vi "Main.vi"() -> ()   [LabVIEW 2020, in "1039_mod.lvlib"]
doc: "This template is based off of the Queued Message Handler design pattern and the Queued Message Handler project template that ships with LabVIEW.\n\nThe main difference is that the queue is private to this module and communication between modules is performed via Broadcast and Request events.\n\nRequest events are wrapped in public API methods and are handled in the Event Handling Loop (EHL) of this VI. Any module can register for Broadcast events sent by this module. The EHL generates messages based on user interface actions.\n\nThe Message Handling Loop (MHL) processes messages generated by the EHL, or by other messages. The messages are string values, so new messages can be added easily to the Message Cases case structure in the MHL. Each message cluster can also provide an optional value for Message Data, which is a variant that can be converted to whatever message-specific data is required.\n_____\nBased on Delacor QMH Project Template 4.2.1.64."
uses:
  1039_mod.lvlib
  <vilib>/Delacor/Delacor QMH/Libraries/Module Admin_class/Delacor_lib_QMH_Module Admin.lvclass
  thcd_controls/ctrl_chn_thcd.ctl
  thcd_controls/ctrl_uom_thcd.ctl
  thcd_controls/ctrl_gid_thcd.ctl
  Module Data--cluster.ctl
  <vilib>/Delacor/Delacor QMH/Libraries/Message Queue_class/Delacor_lib_QMH_Message Queue.lvclass/Delacor_lib_QMH_Message Queue.ctl
  Stop Argument--cluster.ctl
  <vilib>/Delacor/Delacor QMH/Libraries/Module Admin_class/Delacor_lib_QMH_Module Admin.lvclass/Delacor_lib_QMH_Module Admin.ctl
  Initialize Communication Argument--cluster.ctl
  Initialize Instrument Argument--cluster.ctl
  Configure Instrument Argument--cluster.ctl
  Perform Measurement Argument--cluster.ctl
  Perform Measurement (Reply Payload)--cluster.ctl
  <vilib>/Utility/miscctls.llb/LVPointTypeDef.ctl
  <vilib>/Delacor/Delacor QMH/Libraries/Message Queue_class/Delacor_lib_QMH_Enqueue Message (Single).vi
  <vilib>/Delacor/Delacor QMH/Libraries/Module Admin_class/Delacor_lib_QMH_Get External Launch.vi
  <vilib>/Utility/error.llb/Error Cluster From Error Code.vi
  thcd_commands/thcd_set_uom.vi
  thcd_commands/thcd_set_gid.vi
  <vilib>/ErrorRing/Error Ring.xnode
  <vilib>/Delacor/Delacor QMH/Libraries/Message Queue_class/Delacor_lib_QMH_Message Queue.lvclass
panel:
  in  "module_id":u16
  in  "thcd_gid":T1
  in  "thcd_ch":T2
  in  "thcd_uom":T3
  out "thcd_res_1":T4
  in  "dev_baud_rate":u32(ring)=19200 items=["9.6KHz"=9600, "19.2KHz"=19200]
  in  "module_port":refnum<visa-resource-name>
  in  "Simulate MHL Error":bool
  in  "Simulate EHL Error":bool
  out "error out":errorcluster
  in  "Module Admin":refnum<class "Delacor_lib_QMH_Module Admin.lvclass">
  out "Status":string
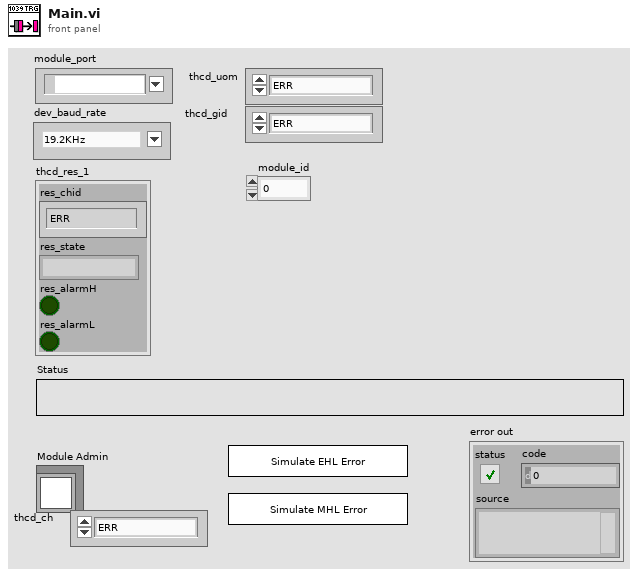
[diagram p1: front panel]
types:
  T1 = typedef "ctrl_gid_thcd.ctl" = enum16{"ERR", "1", "2", "C3H6O_1", "C2H3N", "C2H2", "Air", "C3H4_1", "NH3", "Ar", "AsH3", "C6H6", "BCl3", "BF3", "Br2", "15", "16", "CBrF3", "C4H10_1", "19", "C4H8_1", "CO2", "CS2", "CO", "CCl4", "COS", "Cl2", "ClF3", "28", "29", "CHCl3", "31", "32", "C4H8_2", "C2N2", "ClCN", "C4H8_3", "C3H6", "H22", "B2H6", "40", "R21", "42", "43", "44", "45", "46", "47", "48", "C2H7N_1", "C2H6O_1", "C2H6S_1", "C4H6_1", "C2H6", "54", "55", "C2H6O_2", "C4H6_2", "C2H7N_2", "C8H10", "60", "61", "C2H5F", "C2H4", "64", "65", "C2H4O", "C2H4N", "68", "C2H6S_2", "F2", "CH2O", "CCl3F", "73", "CClF3", "CF4", "76", "CHF3", "78", "C4H4O", "He", "C3HF7", "HMDS", "83", "C6H14", "C6F6", "C6H12_1", "N2H4", "H2", "HBr", "HCl", "CHN", "HF", "HI", "H2Se", "H2S", "C4H10_2", "97", "C4H8_4", "C5H12_1", "C3H8O_1", "101", "C2H2O", "Kr", "CH4", "CH4O", "106", "C3H4_2", "CH5N", "CH3Br", "CH3Cl", "C7H14", "C3H9N", "C3H8O_2", "C3H8S", "CH3F", "116", "CH3I", "CH4S", "C6H12_2", "C3H6O_2", "Ne", "NO", "N2", "NO2", "N2O4", "NF3", "127", "NOCl", "N2O", "C5H12_2", "C8H18", "O2", "F2O", "O3", "B5H9", ""}
  T2 = typedef "ctrl_chn_thcd.ctl" = enum8{"ERR", "1", "2", "3", "4"}
  T3 = typedef "ctrl_uom_thcd.ctl" = enum16{"ERR", "SCCM", "SLM", "%", "V", "MV", "CNT", "NLM", "SLS", "NLS", "SLH", "NLH", "SMLM", "NMLM", "SMLS", "NMLS", "SMLH", "NMLH", "NCCM", "SCCS", "NCCS", "SCCH", "NCCH", "SCFM", "NCFM", "SCFS", "NCFS", "SCFH", "NCFH", "SCMM", "NCMM", "SCMS", "NCMS", "SCMH", "NCMH", "SCIM", "NCIM", "SCIS", "NCIS", "SCIH", "NCIH", "LBM", "LBS", "LBH", "KgM", "KgS", "KgH", "GRM", "GMS", "GRH", "MolM", "MolS", "MolH", "KMolM", "KMolS", "KMolH", "W", "BPS", "Sec", "Min", "Hrs", "WH", "Torr", "Bar", "Pa", "inH2O", "PSIA", "PSIG"}
  T4 = cluster{"res_chid":T2, "res_state":string, "res_alarmH":bool, "res_alarmL":bool}
  T5 = typedef "1039_mod.lvlib/Request Events--cluster.ctl" = cluster{"Stop Module":refnum<user-event>, "Show Panel":refnum<user-event>, "Hide Panel":refnum<user-event>, "Get Module Execution Status":refnum<user-event>, "Show Diagram":refnum<user-event>, "Initialize Communication":refnum<user-event>, "Initialize Instrument":refnum<user-event>, "Configure Instrument":refnum<user-event>, "Perform Measurement":refnum<user-event>}
  T6 = typedef "1039_mod.lvlib/Module Data--cluster.ctl" = cluster{"Status":string}
  T7 = enum32{"invalid lock state", "Not Locked", "Locked (No Password)", "Password-protected"}
  T8 = typedef "1039_mod.lvlib/Stop Argument--cluster.ctl" = cluster{"Origin":string, "Exit via Stop Module Req?":bool, "Wait for Module to stop?":bool}
  T9 = typedef "1039_mod.lvlib/Initialize Communication Argument--cluster.ctl" = cluster{"com_source":enum16{"request argument", "configuration file", "module setting"}, "com_port":refnum<visa-resource-name>}
  T10 = typedef "1039_mod.lvlib/Initialize Instrument Argument--cluster.ctl" = cluster{"status_type":enum16{"status", "value"}}
  T11 = typedef "1039_mod.lvlib/Configure Instrument Argument--cluster.ctl" = cluster{"config_type":enum16{"module setting", "configuration file"}}
  T12 = typedef "1039_mod.lvlib/Perform Measurement Argument--cluster.ctl" = cluster{"read_source":enum16{"request argument", "configuration file", "module setting"}, "Wait Notifier":refnum<notifier>, "wait for reply":bool}
  T13 = typedef "LVPointTypeDef.ctl" = cluster{"Horizontal":i16, "Vertical":i16}
  T14 = enum32{"Invalid", "Standard", "Closed", "Hidden", "Minimized", "Maximized"}
  T15 = typedef "1039_mod.lvlib/Perform Measurement (Reply Payload)--cluster.ctl" = cluster{"module_id":u16, "timestamp":dbl, "value":dbl[], "Perform Measurement_error":errorcluster}
  T16 = enum16{"request argument", "configuration file", "module setting"}
  T17 = cluster{"res_chid":T2, "res_val":dbl, "res_uom":string, "res_gid":string}
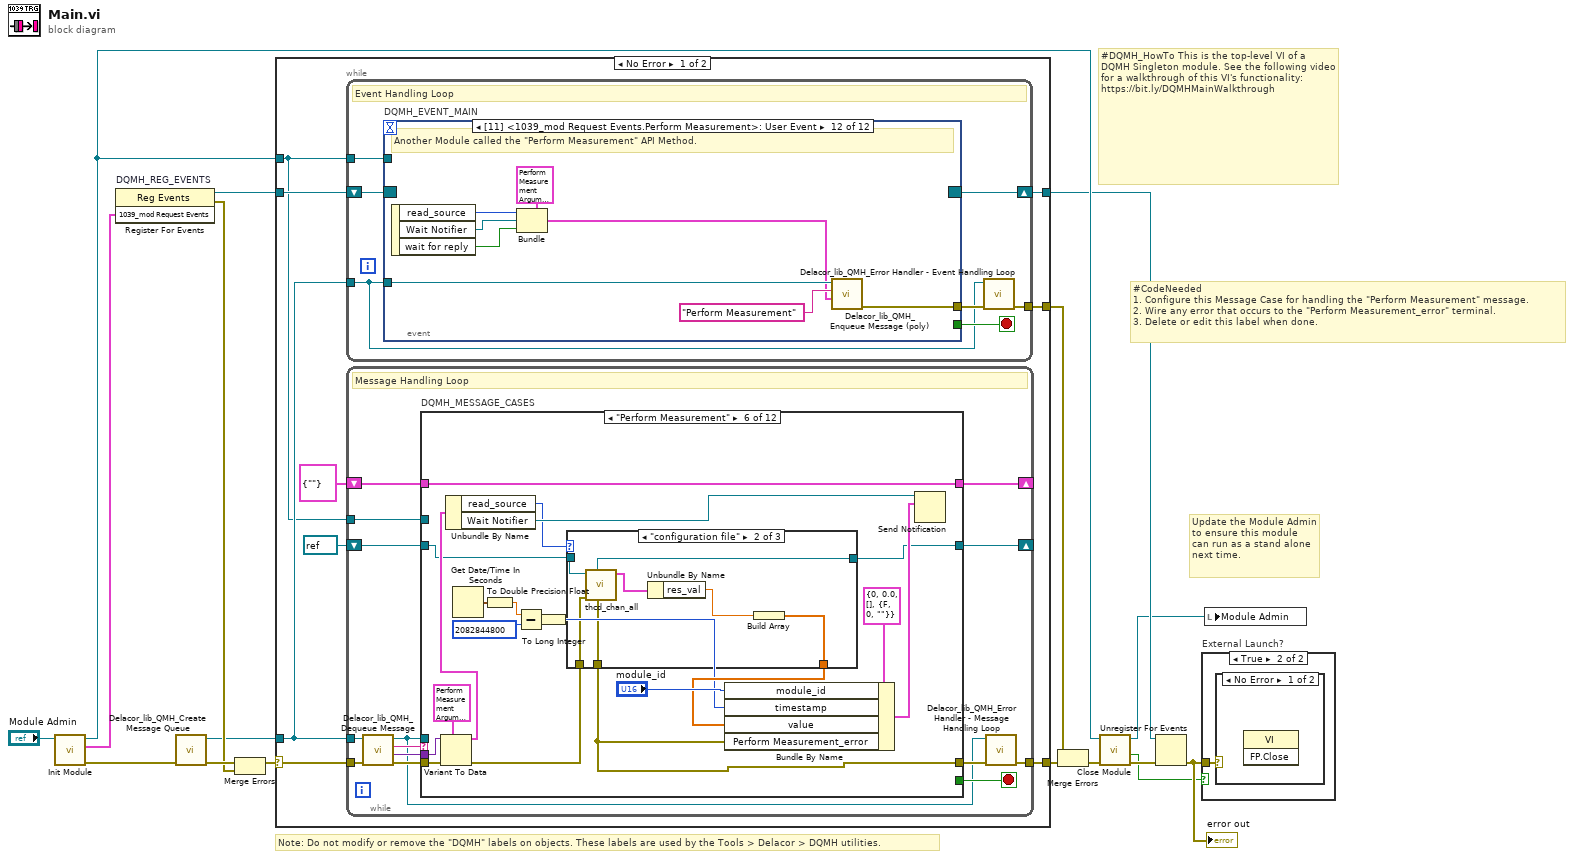
[diagram p0: block diagram]
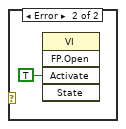
[diagram p3: hidden frame]
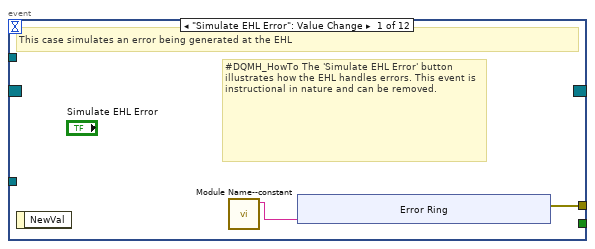
[diagram p4: hidden frame]
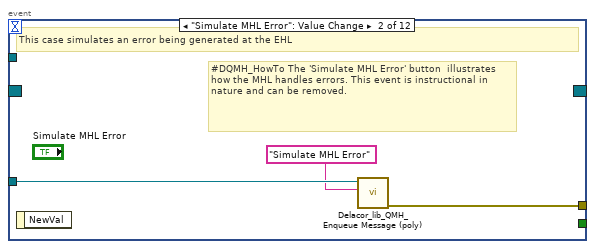
[diagram p5: hidden frame]
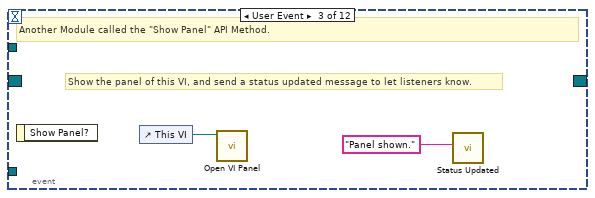
[diagram p6: hidden frame]
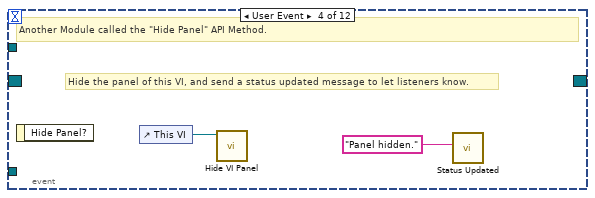
[diagram p7: hidden frame]
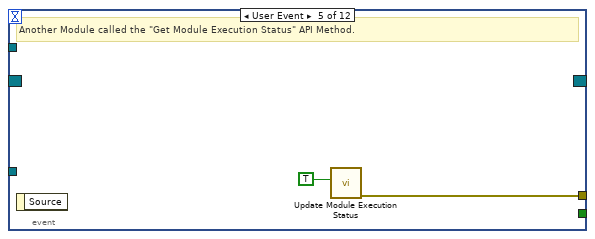
[diagram p8: hidden frame]
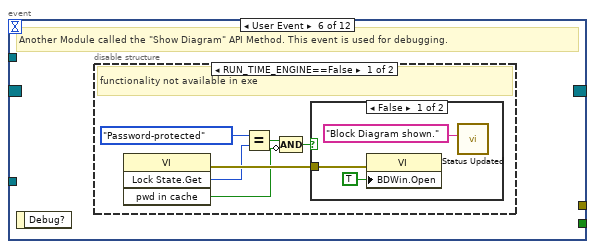
[diagram p9: hidden frame]
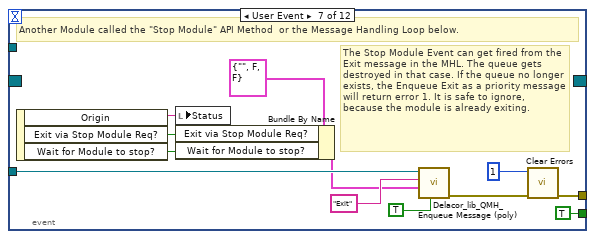
[diagram p12: hidden frame]
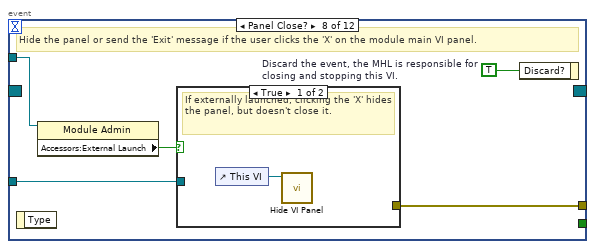
[diagram p13: hidden frame]
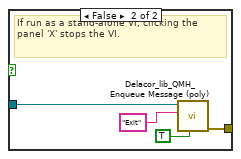
[diagram p14: hidden frame]
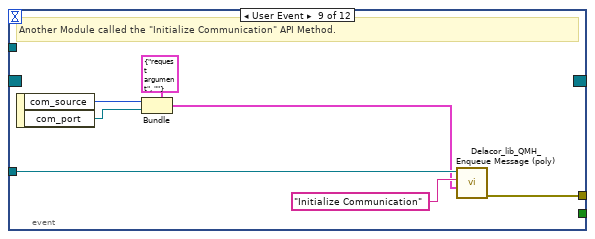
[diagram p15: hidden frame]
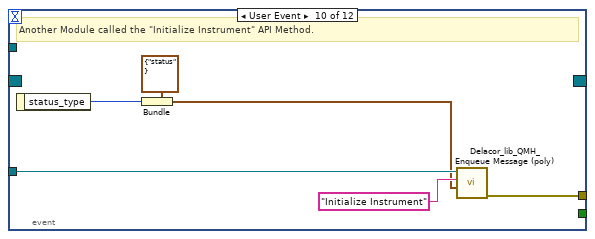
[diagram p16: hidden frame]
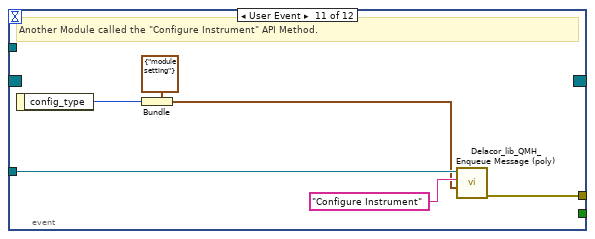
[diagram p17: hidden frame]
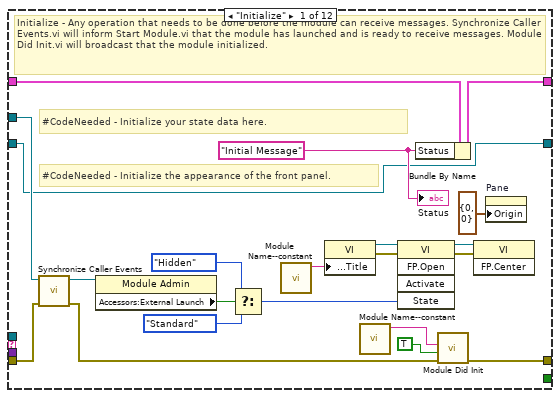
[diagram p18: hidden frame]
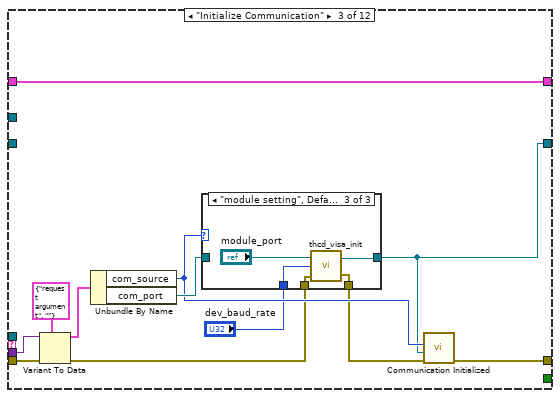
[diagram p20: hidden frame]
diagram:
  # "#CodeNeeded\n1. Configure this Message Case for handling the \"Perform Measurement\" message.\n2. Wire any error that occurs to the \"Perform Measurement_error\" terminal.\n3. Delete or edit this label when done."
  # "#DQMH_HowTo This is the top-level VI of a DQMH Singleton module. See the following video for a walkthrough of this VI's functionality: https://bit.ly/DQMHMainWalkthrough"
  # "Note: Do not modify or remove the \"DQMH\" labels on objects. These labels are used by the Tools > Delacor > DQMH utilities."
  # "Update the Module Admin to ensure this module can run as a stand alone next time."
  n1 = call "Init Module.vi"("Singleton Module Admin in"="Module Admin") -> ("error out"=w16:errorcluster, "1039_mod Request Events"=w5:T5, "Singleton Module Admin out"=w8:refnum<class "Delacor_lib_QMH_Module Admin.lvclass">)  [unwired: 8 in]
  n2 = register-events "DQMH_REG_EVENTS"(w5) -> (reference out=w6:refnum<event-registration>, error out=w9:errorcluster)  [unwired: 2 in]
  n3 = call <vilib>:"Delacor_lib_QMH_Create Message Queue.vi"("error in"=w16) -> ("error out"=w11:errorcluster, "Message Queue"=w4:refnum<class "Delacor_lib_QMH_Message Queue.lvclass">)  [unwired: 9 in]
  n4 = Merge Errors(w11, w9) -> (w10:errorcluster)
  n5 = case shown="No Error" w10 {
    selector: w10 -> [w24 w342]
    tunnel: [w26 w342] -> w17
    tunnel: [w23 w339] -> w7
    tunnel: w6 -> [w21 w339]
    tunnel: w4 -> [w20 _]
    tunnel: [w25 _] -> w14
    tunnel: w8 -> [w19 w335]
    frame No Error {
      n6 = while {
        tunnel: w20 -> [w27]
        shift-right: [w30] -> w23
        shift-left: w21 -> [w31]
        tunnel: [w32] -> w25
        tunnel: w19 -> [w28]
        stop <- w29 stop-if-true
        # "Event Handling Loop"
        n7 = event "DQMH_EVENT_MAIN" shown="[11] <1039_mod Request Events.Perform Measurement>: User Event" {
          selector: w31 -> [_ _ _ _ _ _ _ _ _ _ _ _]
          dyn-events: [_ _ _ _ _ _ _ _ _ _ _ _] -> w30
          timeout: _ -> [_ _ _ _ _ _ _ _ _ _ _ _]
          tunnel: [_ _ _ _ _ _ TRUE ("Discard?") _ _ _ _ _] -> w29
          tunnel: w27 -> [_ w44 _ _ _ _ w68 w75 w89 w95 w101 w109]
          tunnel: [w35 w45 _ _ w51 _ w71 w77 w83 w90 w96 w102] -> w33
          tunnel: w28 -> [_ _ _ _ _ _ _ w74 _ _ _ _]
          event "Simulate EHL Error": Value Change {
            # "#DQMH_HowTo The 'Simulate EHL Error' button  illustrates how the EHL handles errors. This event is instructional in nature and can be removed."
            # "This case simulates an error being generated at the EHL"
            n8 = event-data() -> ()  [unwired: 1 in, 1 out]
            n9 = call "Module Name--constant.vi"() -> ("Module Name"=w34:string)  [unwired: 11 in]
            n10 = xnode "Error Ring"("parameter 0"=w34) -> ("error out"=w35:errorcluster)
          }
          event "Simulate MHL Error": Value Change {
            # "#DQMH_HowTo The 'Simulate MHL Error' button  illustrates how the MHL handles errors. This event is instructional in nature and can be removed."
            # "This case simulates an error being generated at the EHL"
            n11 = event-data() -> ()  [unwired: 1 in, 1 out]
            n12 = call-poly <vilib>:"Delacor_lib_QMH_Enqueue Message (poly).vi"("Message"="Simulate MHL Error", "Message Queue in"=w44) -> ("error out"=w45:errorcluster)  [unwired: 8 in, 1 out]
          }
          event User Event {
            # "Show the panel of this VI, and send a status updated message to let listeners know."
            # "Another Module called the \"Show Panel\" API Method."
            n13 = event-data() -> ()  [unwired: 1 in, 1 out]
            n14 = control-ref of="This VI"() -> (w47:refnum<vi>)
            n15 = call "Open VI Panel.vi"("VI"=w47) -> ()  [unwired: 10 in, 1 out]
            n16 = call "Status Updated.vi"("Status"="Panel shown." ("format string")) -> ()  [unwired: 10 in, 1 out]
          }
          event User Event {
            # "Hide the panel of this VI, and send a status updated message to let listeners know."
            # "Another Module called the \"Hide Panel\" API Method."
            n17 = event-data() -> ()  [unwired: 1 in, 1 out]
            n18 = control-ref of="This VI"() -> (w49:refnum<vi>)
            n19 = call "Hide VI Panel.vi"("VI"=w49) -> ()  [unwired: 10 in, 1 out]
            n20 = call "Status Updated.vi"("Status"="Panel hidden." ("format string")) -> ()  [unwired: 10 in, 1 out]
          }
          event User Event {
            # "Another Module called the \"Get Module Execution Status\" API Method."
            n21 = event-data() -> ()  [unwired: 1 in, 1 out]
            n22 = call "Update Module Execution Status.vi"("Running?"=TRUE) -> ("error out"=w51:errorcluster)  [unwired: 10 in]
          }
          event User Event {
            # "Another Module called the \"Show Diagram\" API Method. This event is used for debugging."
            n23 = event-data() -> ()  [unwired: 1 in, 1 out]
            n24 = disable-structure shown="RUN_TIME_ENGINE==False" {
              frame condition #0 (active) {
                # "functionality not available in exe"
                n25 = invoke class="VI" method="Lock State.Get"() -> (error out=w57:errorcluster, "Get Lock State"=w56:T7, "pwd in cache"=w53:bool)  [unwired: 4 in, 1 out]
                n26 = Equal?(x=T7."Password-protected", y=w56) -> (x = y?=w54:bool)
                n27 = Compound Arithmetic op=AND(w54, invert w53) -> (w52:bool)
                n28 = case shown="False" w52 {
                  tunnel: w57 -> [w60 _]
                  frame False {
                    n29 = property class="VI"(error in=w60, "BDWin.Open"=TRUE ("Block Diagram Window:Open")) -> ()  [unwired: 1 in, 2 out]
                    n30 = call "Status Updated.vi"("Status"="Block Diagram shown." ("format string")) -> ()  [unwired: 10 in, 1 out]
                  }
                  frame True {
                    # "Password-protected VI, and the password is not in the cache. Do not show the diagram."
                  }
                }
              }
              frame condition #1 {
              }
            }
          }
          event User Event {
            # "The Stop Module Event can get fired from the Exit message in the MHL. The queue gets destroyed in that case. If the queue no longer exists, the Enqueue Exit as a priority message will return error 1. It is safe to ignore, because the module is already exiting."
            # "Another Module called the \"Stop Module\" API Method  or the Message Handling Loop below."
            n31 = event-data() -> ("Origin"=w67:string, "Exit via Stop Module Req?"=w63:bool, "Wait for Module to stop?"=w62:bool)  [unwired: 1 in]
            n32 = local write "Status"(w67) -> ()
            n33 = Bundle By Name(cluster=T8 {"Origin"="", "Exit via Stop Module Req?"=FALSE, "Wait for Module to stop?"=FALSE} ("Stop Argument"), "Exit via Stop Module Req?"=w63, "Wait for Module to stop?"=w62) -> (w61:T8)
            n34 = call-poly <vilib>:"Delacor_lib_QMH_Enqueue Message (poly).vi"("Priority Message? (F)"=TRUE, "Message Data"=w61, "Message"="Exit", "Message Queue in"=w68) -> ("error out"=w72:errorcluster)  [unwired: 6 in, 1 out]
            n35 = call <vilib>:"Clear Errors.vi"("error in (no error)"=w72, "specific error code to clear (0: all)"=1) -> ("error out"=w71:errorcluster)  [unwired: 4 in, 1 out]
          }
          event Panel Close? {
            w76 = TRUE  # Discard the event, the MHL is responsible for closing and stopping this VI.
            # "Hide the panel or send the 'Exit' message if the user clicks the 'X' on the module main VI panel."
            n36 = event-data() -> ()  [unwired: 1 in, 1 out]
            n37 = property class="Module Admin"(reference=w74) -> ("Accessors:External Launch"=w73:bool)  [unwired: 1 in, 2 out]
            n38 = case shown="True" w73 {
              tunnel: w75 -> [_ w81]
              tunnel: [_ w82] -> w77
              frame True {
                # "If externally launched, clicking the 'X' hides the panel, but doesn't close it."
                n39 = control-ref of="This VI"() -> (w78:refnum<vi>)
                n40 = call "Hide VI Panel.vi"("VI"=w78) -> ()  [unwired: 10 in, 1 out]
              }
              frame False {
                # "If run as a stand-alone VI, clicking the panel 'X' stops the VI."
                n41 = call-poly <vilib>:"Delacor_lib_QMH_Enqueue Message (poly).vi"("Priority Message? (F)"=TRUE, "Message"="Exit", "Message Queue in"=w81) -> ("error out"=w82:errorcluster)  [unwired: 7 in, 1 out]
              }
            }
            n42 = event-data("Discard?"=w76) -> ()  [unwired: 1 in, 1 out]
          }
          event User Event {
            # "Another Module called the \"Initialize Communication\" API Method."
            n43 = event-data() -> ("com_source"=w85:T16, "com_port"=w84:refnum<visa-resource-name>)  [unwired: 1 in]
            n44 = Bundle(cluster=T9 {"com_source"=enum."request argument", "com_port"=""} ("Initialize Communication Argument"), "com_source"=w85, "com_port"=w84) -> (w86:T9)
            n45 = call-poly <vilib>:"Delacor_lib_QMH_Enqueue Message (poly).vi"("Message Data"=w86, "Message"="Initialize Communication", "Message Queue in"=w89) -> ("error out"=w83:errorcluster)  [unwired: 7 in, 1 out]
          }
          event User Event {
            # "Another Module called the \"Initialize Instrument\" API Method."
            n46 = event-data() -> ("status_type"=w91:enum16{"status", "value"})  [unwired: 1 in]
            n47 = Bundle(cluster=T10 {"status_type"=enum."status"} ("Initialize Instrument Argument"), "status_type"=w91) -> (w92:T10)
            n48 = call-poly <vilib>:"Delacor_lib_QMH_Enqueue Message (poly).vi"("Message Data"=w92, "Message"="Initialize Instrument", "Message Queue in"=w95) -> ("error out"=w90:errorcluster)  [unwired: 7 in, 1 out]
          }
          event User Event {
            # "Another Module called the \"Configure Instrument\" API Method."
            n49 = event-data() -> ("config_type"=w97:enum16{"module setting", "configuration file"})  [unwired: 1 in]
            n50 = Bundle(cluster=T11 {"config_type"=enum."module setting"} ("Configure Instrument Argument"), "config_type"=w97) -> (w98:T11)
            n51 = call-poly <vilib>:"Delacor_lib_QMH_Enqueue Message (poly).vi"("Message Data"=w98, "Message"="Configure Instrument", "Message Queue in"=w101) -> ("error out"=w96:errorcluster)  [unwired: 7 in, 1 out]
          }
          event User Event {
            # "Another Module called the \"Perform Measurement\" API Method."
            n52 = event-data() -> ("read_source"=w105:T16, "Wait Notifier"=w104:refnum<notifier>, "wait for reply"=w103:bool)  [unwired: 1 in]
            n53 = Bundle(cluster=T12 {"read_source"=enum."request argument", "Wait Notifier"=refnum, "wait for reply"=FALSE} ("Perform Measurement Argument"), "read_source"=w105, "Wait Notifier"=w104, "wait for reply"=w103) -> (w106:T12)
            n54 = call-poly <vilib>:"Delacor_lib_QMH_Enqueue Message (poly).vi"("Message Data"=w106, "Message"="Perform Measurement", "Message Queue in"=w109) -> ("error out"=w102:errorcluster)  [unwired: 7 in, 1 out]
          }
        }
        n55 = call-dynamic "Delacor_lib_QMH_Error Handler - Event Handling Loop.vi"("error in"=w33, "Message Queue in"=w27) -> ("dup error in"=w32:errorcluster)  [unwired: 8 in, 1 out]
      }
      n56 = while {
        tunnel: w20 -> [w114]
        shift-right: [w118] -> _
        shift-left: T6 {"Status"=""} ("Data Cluster") -> [w119]
        tunnel: w24 -> [w122]
        tunnel: [w120] -> w26
        tunnel: w19 -> [w112]
        shift-right: [w111] -> _
        shift-left: refnum<visa-resource-name> refnum ("module_port") -> [w110]
        stop <- w117 stop-if-true
        # "Message Handling Loop"
        n57 = call-dynamic "Delacor_lib_QMH_Dequeue Message.vi"("error in"=w122, "Message Queue in"=w114) -> ("error out"=w121:errorcluster, "Message Data"=w115:variant, "Message"=w116:string, "Message Queue out"=w113:refnum<class "Delacor_lib_QMH_Message Queue.lvclass">)  [unwired: 6 in]
        n58 = case "DQMH_MESSAGE_CASES" shown="\"Perform Measurement\"" w116 {
          selector: w116 -> [_ _ _ _ _ _ _ _ _ _ _ w322]
          tunnel: w113 -> [_ _ _ _ _ _ _ _ _ w290 w313 _]
          tunnel: w121 -> [w142 w147 w159 w181 w210 w246 w270 w273 w279 w297 w319 w324]
          tunnel: [w140 w147 w153 w170 w194 w232 w269 w273 w278 w293 w316 w325] -> w123
          tunnel: w119 -> [w131 w146 w158 w180 w209 w245 w268 w272 w276 w292 w312 w323]
          tunnel: [w130 w146 w158 w180 w209 w245 w268 w272 w276 w292 w312 w323] -> w118
          tunnel: [_ _ _ _ _ _ _ _ _ _ w311 _] -> w117
          tunnel: w115 -> [_ _ w157 w179 w208 w244 _ _ _ w291 w310 _]
          tunnel: w112 -> [w132 _ _ _ _ _ _ _ _ w289 w305 _]
          tunnel: [w124 w145 w148 w174 w200 w236 w267 w271 w274 w287 w304 w320] -> w111
          tunnel: w110 -> [w124 w145 _ w175 w204 w237 w267 w271 w274 w287 w304 w320]
          frame "Initialize" {
            w125 = "Initial Message" ("Initial Message")
            # "#CodeNeeded - Initialize the appearance of the front panel."
            # "#CodeNeeded - Initialize your state data here."
            # "Initialize - Any operation that needs to be done before the module can receive messages. Synchronize Caller Events.vi will inform Start Module.vi that the module has launched and is ready to receive messages. Module Did Init.vi will broadcast that the module initialized."
            n59 = call "Synchronize Caller Events.vi"("error in (no error)"=w142, "Singleton Module Admin in"=w132) -> ("error out"=w141:errorcluster, "Singleton Module Admin out"=w127:refnum<class "Delacor_lib_QMH_Module Admin.lvclass">)  [unwired: 8 in]
            n60 = property class="Module Admin"(reference=w127) -> ("Accessors:External Launch"=w136:bool)  [unwired: 1 in, 2 out]
            n61 = Select(t=T14."Hidden" ("State"), s=w136, f=T14."Standard" ("State")) -> (s? t:f=w133:T14)
            n62 = call "Module Name--constant.vi"() -> ("Module Name"=w139:string)  [unwired: 11 in]
            n63 = property class="VI"("Front Panel.Title"=w139) -> (reference out=w138:refnum<vi>, error out=w144:errorcluster)  [unwired: 2 in]
            n64 = call "Module Name--constant.vi"() -> ("Module Name"=w128:string)  [unwired: 11 in]
            n65 = invoke class="VI" method="FP.Open"(reference=w138, error in=w144, "State"=w133) -> (reference out=w137:refnum<vi>, error out=w143:errorcluster)  [unwired: 2 in, 3 out]
            n66 = Bundle By Name(cluster=w131, "Status"=w125) -> (w130:T6)
            n67 = call "Module Did Init.vi"("error in (no error)"=w141, "Initialized?"=TRUE, "Origin"=w128) -> ("error out"=w140:errorcluster)  [unwired: 8 in]
            n68 = invoke class="VI" method="FP.Center"(reference=w137, error in=w143) -> ()  [unwired: 1 in, 3 out]
            n69 = property on="Pane" class="Pane"("Origin"=T13 {"Horizontal"=0, "Vertical"=0}) -> ()  [unwired: 2 in, 2 out]
            "Status" <- w125
          }
          frame "--- Module Specific ---" {
            # "Separator -- The following cases handle messages specific to this Module."
          }
          frame "Initialize Communication" {
            n70 = Variant To Data(error in=w159, type=T9 {"com_source"=enum."request argument", "com_port"=""} ("Initialize Communication Argument"), Variant=w157) -> (data=w155:T9, error out=w150:errorcluster)
            n71 = Unbundle By Name(w155) -> ("com_source"=w152:T16, "com_port"=w154:refnum<visa-resource-name>)
            n72 = case shown="\"module setting\", Default" w152 {
              tunnel: [w161 refnum<visa-resource-name> refnum ("module_port") w167] -> w148
              tunnel: w154 -> [w161 _ _]
              tunnel: "dev_baud_rate" -> [_ _ w166]
              tunnel: w150 -> [w160 w162 w165]
              tunnel: [w160 w162 w164] -> w149
              frame "request argument" {
              }
              frame "configuration file" {
              }
              frame "module setting", Default {
                n73 = call "thcd_visa_init.vi"("err_in"=w165, "Serial Settings:Baud Rate"=w166, "thcd_visa"="module_port") -> ("err_out"=w164:errorcluster, "thcd_visa"=w167:refnum<visa-resource-name>)
              }
            }
            n74 = call "Communication Initialized.vi"("error in (no error)"=w149, "com_port"=w148, "com_source"=w152) -> ("error out"=w153:errorcluster)  [unwired: 8 in]
          }
          frame "Initialize Instrument" {
            n75 = Variant To Data(error in=w181, type=T10 {"status_type"=enum."status"} ("Initialize Instrument Argument"), Variant=w179) -> (data=w177:T10, error out=w173:errorcluster)
            n76 = Unbundle By Name(w177) -> ("status_type"=w176:enum16{"status", "value"})
            n77 = case shown="\"status\", Default" w176 {
              tunnel: w175 -> [w189 w192]
              tunnel: [w188 w192] -> w174
              tunnel: w173 -> [w187 w191]
              tunnel: [w184 w191] -> w171
              tunnel: [w183 T4 {"res_chid"=enum."1", "res_state"="ok", "res_alarmH"=TRUE, "res_alarmL"=TRUE} ("thcd_res_1")] -> w172
              tunnel: [w182 TRUE ("thcd_st")] -> w169
              frame "status", Default {
                n78 = call "thcd_chan_stat.vi"("err_in"=w187, "thcd_b2r"=u32 300, "thcd_delay"=u32 300, "thcd_visa"=w189) -> ("thcd_res_1"=w183:T4, "thcd_st"=w182:bool, "err_out"=w184:errorcluster, "thcd_visa"=w188:refnum<visa-resource-name>)  [unwired: 4 out]
              }
              frame "value" {
              }
            }
            "thcd_res_1" <- w172
            n79 = call "Instrument Initialized.vi"("error in (no error)"=w171, "instr_status"=w169) -> ("error out"=w170:errorcluster)  [unwired: 9 in]
          }
          frame "Configure Instrument" {
            n80 = Variant To Data(error in=w210, type=T11 {"config_type"=enum."module setting"} ("Configure Instrument Argument"), Variant=w208) -> (data=w206:T11, error out=w201:errorcluster)
            n81 = Unbundle By Name(w206) -> ("config_type"=w205:enum16{"module setting", "configuration file"})
            n82 = case shown="\"configuration file\"" w205 {
              tunnel: w204 -> [w221 w226]
              tunnel: "thcd_uom" -> [w212 w224]
              tunnel: "thcd_ch" -> [w218 _]
              tunnel: w201 -> [w217 w225]
              tunnel: [w216 w226] -> w200
              tunnel: "thcd_gid" -> [w213 w223]
              tunnel: [w214 w225] -> w196
              tunnel: [w212 w224] -> w198
              tunnel: [w213 w223] -> w197
              tunnel: [w211 TRUE ("thcd_st")] -> w195
              frame "module setting", Default {
                n83 = call-poly "thcd_setters.vi"("thcd_delay"=u32 500, "err_in"=w217, "thcd_val"=w212, "thcd_ch"=w218, "thcd_visa"=w221) -> ("err_out"=w215:errorcluster, "thcd_visa"=w219:refnum<visa-resource-name>)  [unwired: 1 in, 2 out]
                n84 = call-poly "thcd_setters.vi"("err_in"=w215, "thcd_val"=w213, "thcd_ch"=w218, "thcd_visa"=w219) -> ("err_out"=w214:errorcluster, "thcd_st"=w211:bool, "thcd_visa"=w216:refnum<visa-resource-name>)  [unwired: 2 in, 1 out]
              }
              frame "configuration file" {
              }
            }
            n85 = call "Instrument Configured.vi"("config_stat"=w195, "error in (no error)"=w196, "config_set2"=w197, "config_set1"=w198) -> ("error out"=w194:errorcluster)  [unwired: 7 in]
          }
          frame "Perform Measurement" {
            n86 = Variant To Data(error in=w246, type=T12 {"read_source"=enum."request argument", "Wait Notifier"=refnum, "wait for reply"=FALSE} ("Perform Measurement Argument"), Variant=w244) -> (data=w242:T12, error out=w233:errorcluster)
            n87 = Unbundle By Name(w242) -> ("read_source"=w238:T16, "Wait Notifier"=w241:refnum<notifier>)
            n88 = Get Date/Time In Seconds() -> (seconds since 1Jan1904=w229:timestamp)
            n89 = To Double Precision Float(number=w229) -> (double precision float=w231:dbl)
            n90 = Subtract(x=w231, y=2082844800 ("01Jan1970, UTC")) -> (x-y=w230:dbl)
            n91 = To Long Integer(number=w230) -> (32bit integer=w227:i32)
            n92 = case shown="\"configuration file\"" w238 {
              tunnel: w237 -> [w248 w256 w258]
              tunnel: [w248 w255 w258] -> w236
              tunnel: [dbl[] [] w250 w259] -> w234
              tunnel: [w247 w254 w257] -> w232
              tunnel: w233 -> [w247 w253 w257]
              frame "request argument", Default {
              }
              frame "configuration file" {
                n93 = call "thcd_chan_all.vi"("err_in"=w253, "thcd_visa"=w256) -> ("thcd_res_1"=w252:T17, "err_out"=w254:errorcluster, "thcd_visa"=w255:refnum<visa-resource-name>)  [unwired: 5 in, 2 out]
                n94 = Unbundle By Name(w252) -> ("res_val"=w251:dbl)
                n95 = Build Array(w251) -> (w250:dbl[])
              }
              frame "module setting" {
                n96 = for {
                  N: 3 -> [_]
                  tunnel: [w261] -> w259 mode=indexing
                  i -> [w264]
                  n97 = Random Number (0-1)() -> (number: 0 to 1=w266:dbl)
                  n98 = Increment(x=w264) -> (x+1=w263:i32)
                  n99 = Multiply(x=10.0, y=w263) -> (x*y=w262:dbl)
                  n100 = Add(x=w266, y=w262) -> (x+y=w261:dbl)
                }
              }
            }
            n101 = Bundle By Name(cluster=T15 {"module_id"=0, "timestamp"=0.0, "value"=[], "Perform Measurement_error"={"status"=FALSE, "code"=0, "source"=""}} ("Perform Measurement (Reply Payload)"), "module_id"="module_id", "timestamp"=w227, "value"=w234, "Perform Measurement_error"=w232) -> (w240:T15)
            n102 = Send Notification(notification=w240, notifier=w241) -> ()  [unwired: 1 in, 2 out]
          }
          frame "---Copy This Frame---" {
            # "Duplicate this frame when creating new messages.  Change this comment in the duplicated frame to describe this message."
            n103 = Merge Errors(w270) -> (w269:errorcluster)
          }
          frame "--- Exit and Error Handling---" {
            # "Separator - The following cases handle errors and exit messages."
          }
          frame "Simulate MHL Error" {
            # "#DQMH_HowTo The 'Simulate MHL Error' button  illustrates how the MHL handles errors. This event is instructional in nature and can be removed."
            # "Simulate an error occurring at the MHL"
            n104 = call "Module Name--constant.vi"() -> ("Module Name"=w275:string)  [unwired: 11 in]
            n105 = xnode "Error Ring"("parameter 0"=w275) -> ("error out"=w277:errorcluster)
            n106 = Merge Errors(w279, w277) -> (w278:errorcluster)
          }
          frame "Error" {
            # "#CodeRecommended - If you ever change the name of this \"Error\" message, you'll need to update the name in the Check Loop Error.vi as well."
            # "#CodeRecommended - If the module is running in standalone mode (External Launch = FALSE), this code will pop up an error dialog and call the 'Exit' message if an error occurs. Add more fine-grained error handling here."
            # "Error - Check the error message data and respond accordingly. This message is sent by the \"Error Handler\" VIs at the end of each loop in this application."
            n107 = property class="Module Admin"(reference=w289) -> ("Accessors:External Launch"=w288:bool)  [unwired: 1 in, 2 out]
            n108 = Variant To Data(error in=w297, type=errorcluster {"status"=FALSE, "code"=0, "source"=""} ("error constant"), Variant=w291) -> (data=w298:errorcluster, error out=w295:errorcluster)
            n109 = call "Error Reported.vi"("Error"=w298) -> ()  [unwired: 10 in, 1 out]
            n110 = case shown="False" w288 {
              tunnel: [w303 _] -> w294
              tunnel: w290 -> [w301 _]
              tunnel: w298 -> [w302 _]
              frame False {
                # "If the module is running standalone, then pop up an error dialog and call the \"Exit\" message."
                n111 = call <vilib>:"Simple Error Handler.vi"("error in (no error)"=w302) -> ()  [unwired: 4 in, 5 out]
                n112 = call-poly <vilib>:"Delacor_lib_QMH_Enqueue Message (poly).vi"("Priority Message? (F)"=TRUE, "Message"="Exit", "Message Queue in"=w301) -> ("error out"=w303:errorcluster)  [unwired: 7 in, 1 out]
              }
              frame True {
                # "If the module was launched externally, calling the Error Reported broadcast VI is the only action performed by the \"Error\" message. The module's caller can then process the error appropriately."
              }
            }
            n113 = Merge Errors(w295, w294) -> (w293:errorcluster)
            n114 = local write "error out"(w293) -> ()
          }
          frame "Exit" {
            w309 = 91  # 91: not all Exit messages will have an argument
            w311 = TRUE  # Stop the VI
            # "Release the message queue reference"
            # "#CodeNeeded - Add any required cleanup code here"
            # "Exit - Exit the application."
            n115 = Variant To Data(error in=w319, type=T8 {"Origin"="", "Exit via Stop Module Req?"=FALSE, "Wait for Module to stop?"=FALSE} ("Stop Argument"), Variant=w310) -> (data=w307:T8, error out=w315:errorcluster)
            n116 = call <vilib>:"Clear Errors.vi"("error in (no error)"=w315, "specific error code to clear (0: all)"=w309) -> ("error out"=w318:errorcluster)  [unwired: 4 in, 1 out]
            n117 = control-ref of="This VI"() -> (w306:refnum<vi>)
            n118 = call-dynamic "Delacor_lib_QMH_Release Message Queue.vi"("error in"=w318, "Message Queue"=w313) -> ("error out"=w317:errorcluster)  [unwired: 9 in]
            n119 = call "Handle Exit.vi"("Stop Argument"=w307, "Admin in"=w305, "VI reference"=w306) -> ("error out"=w314:errorcluster)  [unwired: 7 in, 1 out]
            n120 = Merge Errors(w317, w314) -> (w316:errorcluster)
          }
          frame Default {
            # "'Default' case only runs if there is a message that isn't defined in any of the other cases.  Output a programming error."
            n121 = call "Module Name--constant.vi"() -> ("Module Name"=w321:string)  [unwired: 11 in]
            n122 = xnode "Error Ring"("parameter 0"=w322, "parameter 1"=w321) -> ("error out"=w326:errorcluster)
            n123 = Merge Errors(w324, w326) -> (w325:errorcluster)
          }
        }
        n124 = call-dynamic "Delacor_lib_QMH_Error Handler - Message Handling Loop.vi"("error in"=w123, "Message Queue in"=w113) -> ("dup error in"=w120:errorcluster)  [unwired: 8 in, 1 out]
      }
    }
    frame Error {
      # "Synchronize Caller Events.vi will inform Start Module.vi that the module has launched and will let the code calling Start Module.vi register for broadcasts and would permit the caller receive the broadcast that an error occurred at launch time."
      n125 = call "Synchronize Caller Events.vi"("Singleton Module Admin in"=w335) -> ("error out"=w340:errorcluster)  [unwired: 9 in, 1 out]
      n126 = call "Module Name--constant.vi"() -> ("Module Name"=w338:string)  [unwired: 11 in]
      n127 = Format Into String(format string="An error occurred during initialization. %s is no longer running.", w338) -> (resulting string=w336:string)  [unwired: 2 in, 1 out]
      n128 = Merge Errors(w342, w340) -> (w341:errorcluster)
      n129 = call "Error Reported.vi"("Additional Information"=w336, "Error"=w341) -> ()  [unwired: 9 in, 1 out]
    }
  }
  n130 = Merge Errors(w14, w17) -> (w13:errorcluster)
  n131 = call "Close Module.vi"("error in (no error)"=w13, "Module Admin in"=w8) -> ("error out"=w15:errorcluster, "External Launch"=w1:bool, "Module Admin out"=w2:refnum<class "Delacor_lib_QMH_Module Admin.lvclass">)  [unwired: 7 in]
  n132 = Unregister For Events(event registration refnum=w7, error in=w15) -> (error out=w12:errorcluster)
  "error out" <- w12
  n133 = case "External Launch?" shown="True" w1 {
    tunnel: w12 -> [_ w343]
    frame False {
    }
    frame True {
      n134 = case shown="No Error" w343 {
        frame No Error {
          n135 = invoke class="VI" method="FP.Close"() -> ()  [unwired: 3 in, 3 out]
        }
        frame Error {
          n136 = invoke class="VI" method="FP.Open"("Activate"=TRUE ("Activate?")) -> ()  [unwired: 4 in, 5 out]
        }
      }
    }
  }
  n137 = local write "Module Admin"(w2) -> ()
